vi "Periodic Tasks.vi"() -> ()   [LabVIEW 2011]
doc: "This VI runs in parallel to other tasks. It can contain as many user-defined periodic loops as you need. These can carry out PID or other sorts of timed response."
uses:
  <vilib>/Rock Robotics/WPI/Relay/WPI_RelayValue.ctl
  <vilib>/Rock Robotics/SystemInterfaces/Utilities/FPGA_UtilitiesLED State.ctl
  <vilib>/Rock Robotics/SystemInterfaces/Utilities/FPGA_UtilitiesLED Source.ctl
  Robot Global Data.vi
panel:
  out "Distance 2":dbl
  out "Direction 2":bool
  out "error out 3":errorcluster
  out "Rate 2":dbl
  out "Rate":dbl
  out "error out 2":errorcluster
  out "error out":errorcluster
  out "I2C":bool
  out "Heading 2":u16
  out "loop time":u32
  out "Angular Rate":dbl
  out "Angle":dbl
  out "Direction":bool
  out "Distance":dbl
  in  "Home Speed":dbl=1.0
  in  "Home Position":dbl=2.85
  out "Current Voltage":dbl
  in  "upper limit":dbl=4.5
  in  "lower limit":dbl=0.85
  # "Speed to move to home"
  # "Target Tracking"
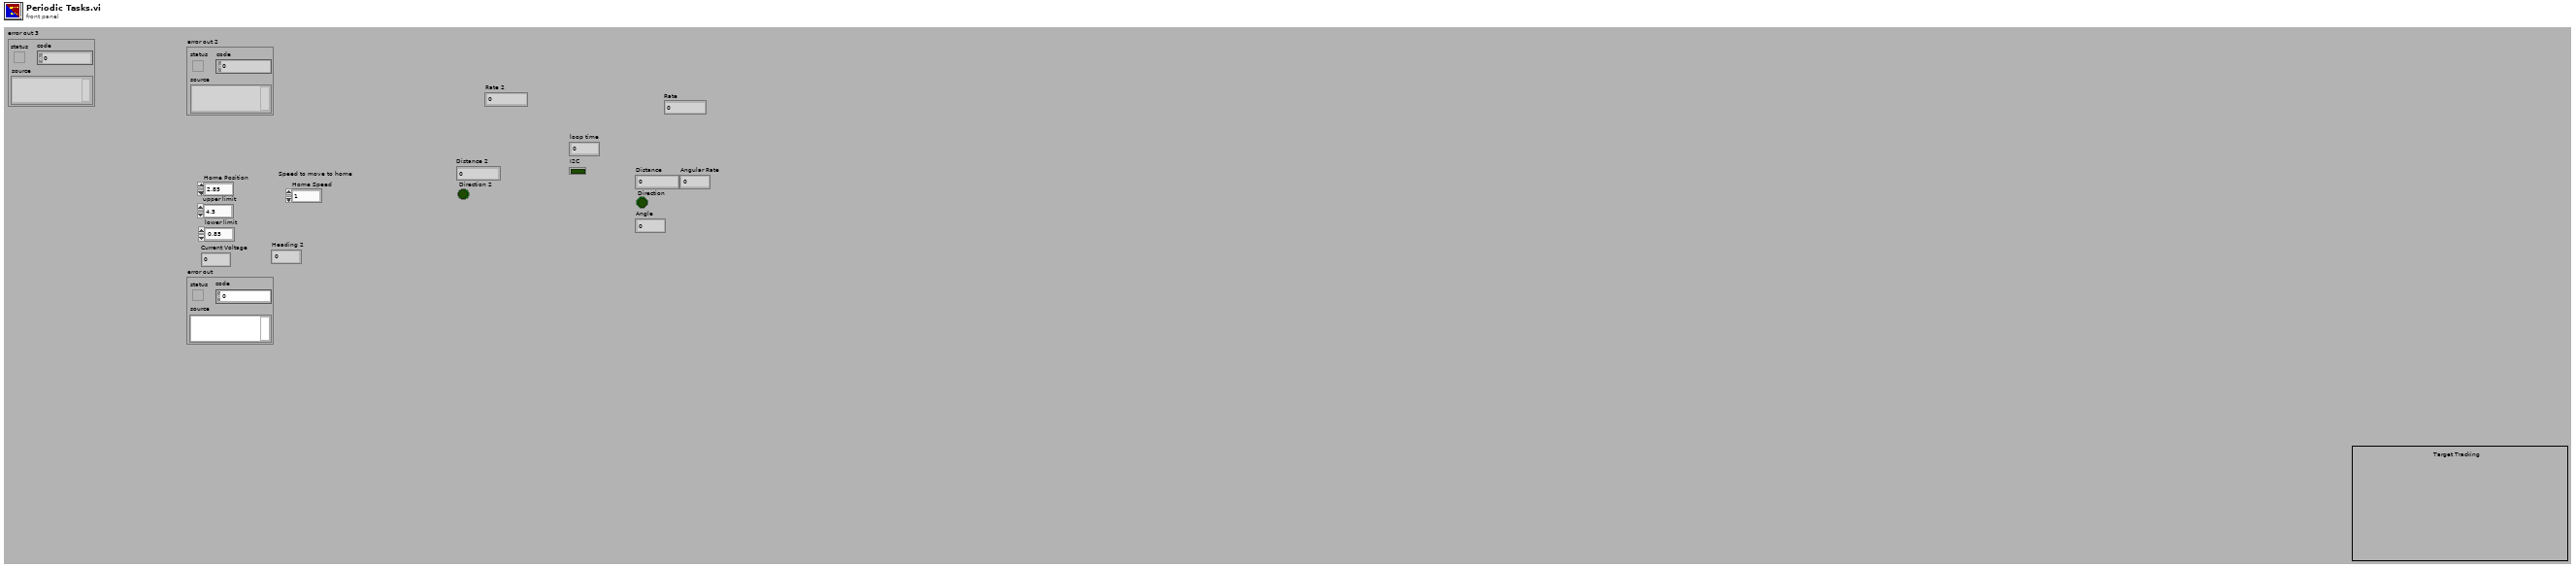
[diagram p1: front panel]
types:
  T1 = typedef "WPI_EncoderDevRef.ctl" = cluster{"DevStatus":errorcluster, "EncoderIndex":T2, "CounterIndex":T3, "DistancePerCount":dbl, "Decoding Type":T4}
  T2 = typedef "FPGA_EncoderIdx.ctl" = enum8{"Enc 0", "Enc 1", "Enc 2", "Enc 3", "Invalid"}
  T3 = typedef "FPGA_CounterCtrSystemIndex.ctl" = enum8{"Ctr 0", "Ctr 1", "Ctr 2", "Ctr 3", "Ctr 4", "Ctr 5", "Ctr 6", "Ctr 7", "Invalid"}
  T4 = typedef "WPI_EncoderType.ctl" = enum16{"1x", "2x", "4x"}
  T5 = typedef "WPI_RelayValue.ctl" = enum16{"Off", "On", "Forward", "Reverse"}
  T6 = typedef "WPI_GyroDevRef.ctl" = cluster{"DevStatus":errorcluster, "Analog Module":T7, "Analog Channel":T8, "Offset":dbl, "Gain (VoltsPerDegree/Second)":dbl}
  T7 = typedef "FPGA_TypedefAnalogModule.ctl" = enum16{"Analog Module 1", "Analog Module 2"}
  T8 = typedef "FPGA_AIChannel.ctl" = enum8{"AI 1", "AI 2", "AI 3", "AI 4", "AI 5", "AI 6", "AI 7", "AI 8", "Invalid"}
  T9 = typedef "WPI_I2CDevRef.ctl" = cluster{"DevStatus":errorcluster, "Digital Module":T10, "Device Address":u8}
  T10 = typedef "FPGA_TypedefDigitalModule.ctl" = enum16{"Digital Module 1", "Digital Module 2"}
  T11 = typedef "WPI_AnalogChannelDevRef.ctl" = cluster{"DevStatus":errorcluster, "Analog Module":T7, "Analog Channel":T8}
  T12 = typedef "WPI_RelayDevRef.ctl" = cluster{"DevStatus":errorcluster, "Relay Channel":T13, "Digital Module":T10, "Relay Direction":T14}
  T13 = typedef "FPGA_DIORelayChannel.ctl" = enum8{"Relay 1", "Relay 2", "Relay 3", "Relay 4", "Relay 5", "Relay 6", "Relay 7", "Relay 8", "Invalid"}
  T14 = typedef "WPI_RelayDirection.ctl" = enum16{"Both directions", "Forward only", "Reverse only"}
  T15 = cluster{"Driver Station Digital Output (1-8)[0]":bool, "Driver Station Digital Output (1-8)[1]":bool, "Driver Station Digital Output (1-8)[2]":bool, "Driver Station Digital Output (1-8)[3]":bool, "Driver Station Digital Output (1-8)[4]":bool, "Driver Station Digital Output (1-8)[5]":bool, "Driver Station Digital Output (1-8)[6]":bool, "Driver Station Digital Output (1-8)[7]":bool, "Driver Station Digital Output (1-8)[8]":bool}
  T16 = typedef "FPGA_UtilitiesLED State.ctl" = enum16{"Off", "On", "Toggle"}
  T17 = typedef "FPGA_UtilitiesLED Source.ctl" = enum16{"User LED", "FPGA LED"}
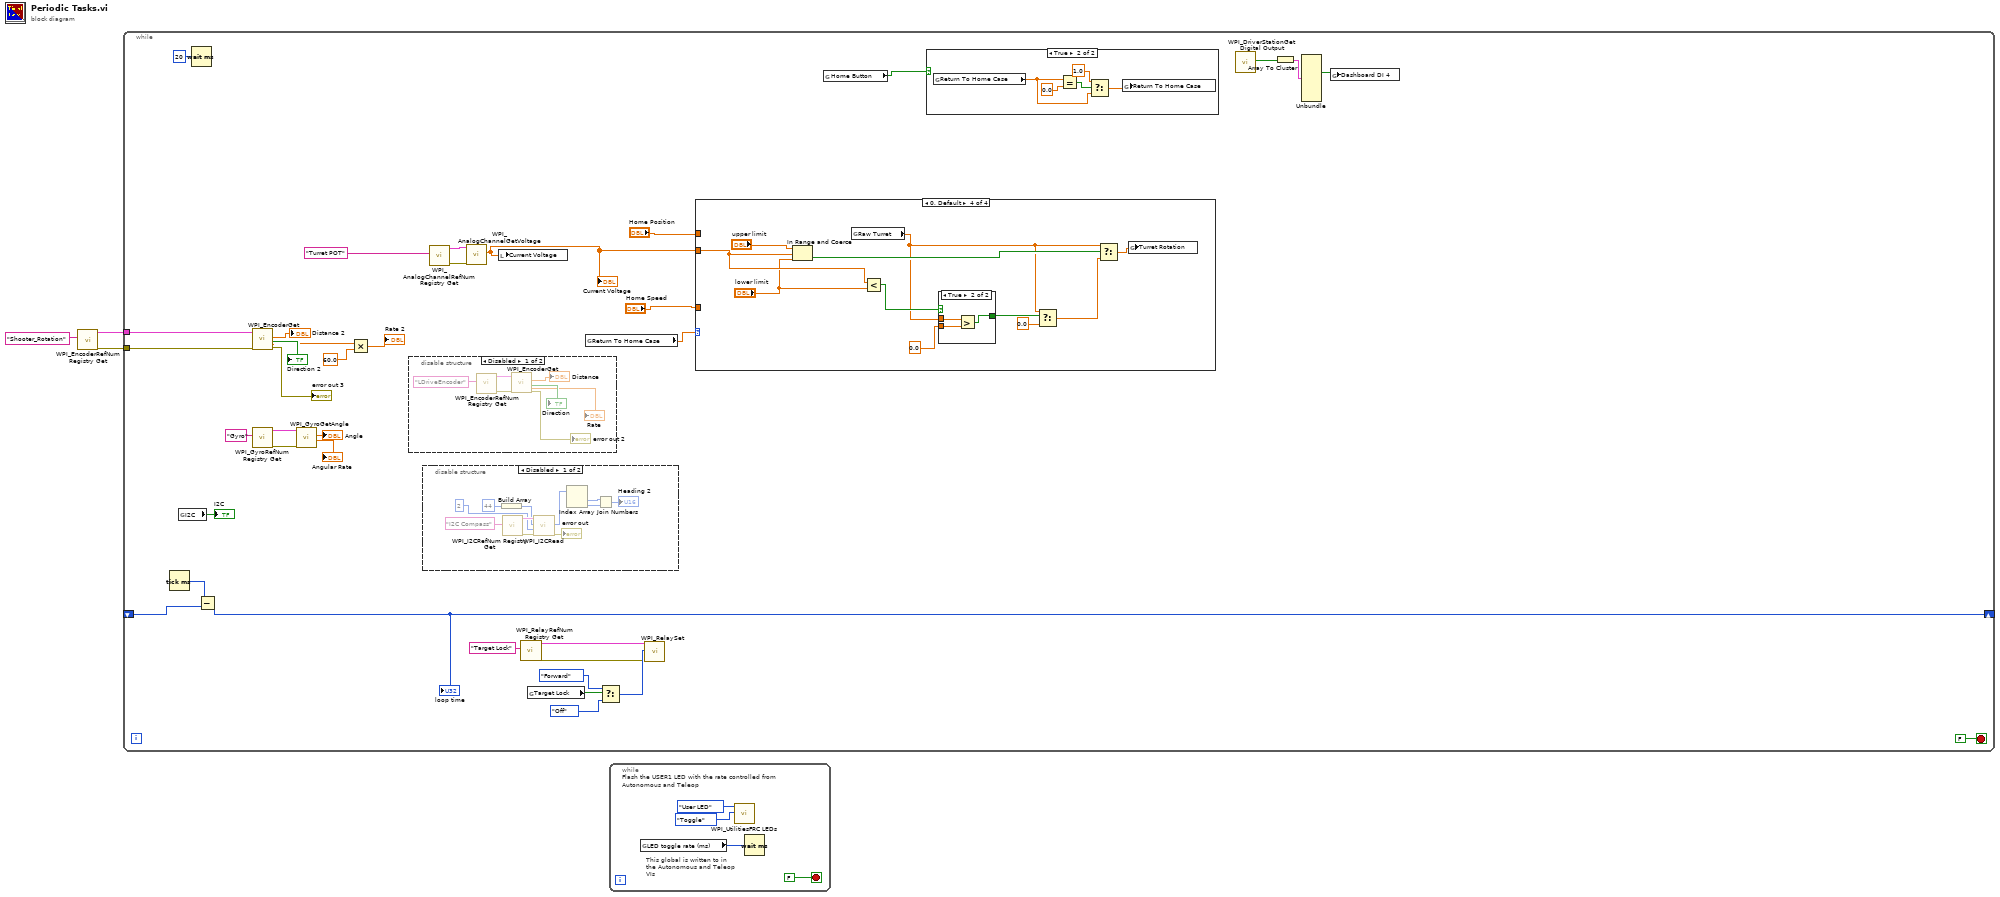
[diagram p0: block diagram]
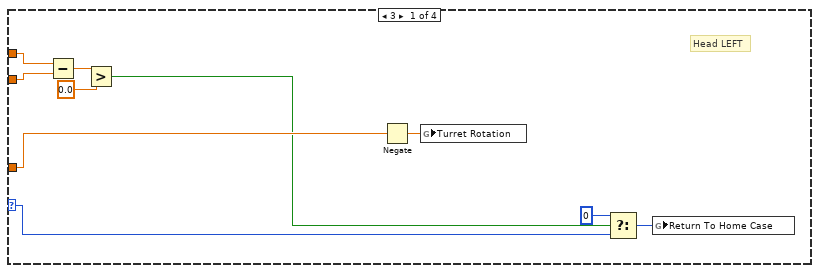
[diagram p4: hidden frame]
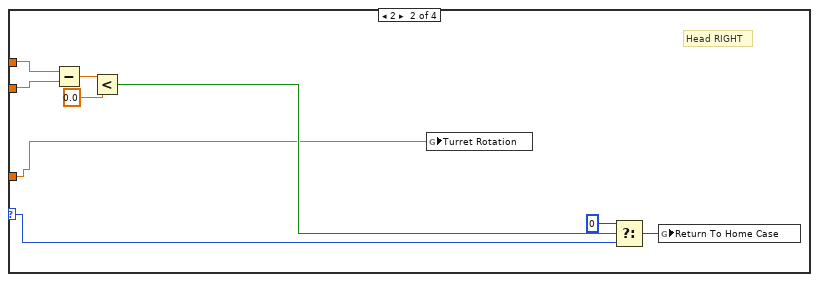
[diagram p5: hidden frame]
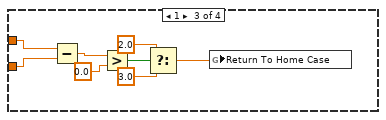
[diagram p6: hidden frame]
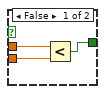
[diagram p7: hidden frame]
diagram:
  n1 = call <vilib>:"WPI_EncoderRefNum Registry Get.vi"("refnum name"="Shooter_Rotation") -> ("error out"=w2:errorcluster, "EncoderDevRef"=w1:T1)  [unwired: 9 in]
  n2 = while {
    shift-right: [w14] -> _
    shift-left: _ -> [w13]
    tunnel: w2 -> [w8]
    tunnel: w1 -> [w7]
    stop <- FALSE stop-if-true
    n3 = Tick Count (ms)() -> (millisecond timer value=w15:u32)
    n4 = global read "Robot Global Data.vi" "I2C"() -> (→"I2C":bool)
    n5 = Wait (ms)(milliseconds to wait=u32 20) -> ()  [unwired: 1 out]
    n6 = Subtract(x=w15, y=w13) -> (x-y=w14:u32)
    "loop time" <- w14
    n7 = call <vilib>:"WPI_EncoderGet.vi"("error in (no error)"=w8, "EncoderDevRef"=w7) -> ("error out"=→"error out 3":errorcluster, "Direction"=→"Direction 2":bool, "Distance"=→"Distance 2":dbl, "Rate"=w5:dbl)  [unwired: 4 in, 2 out]
    n8 = call <vilib>:"WPI_GyroRefNum Registry Get.vi"("refnum name"="Gyro") -> ("error out"=w19:errorcluster, "GyroDevRef"=w20:T6)  [unwired: 9 in]
    n9 = call <vilib>:"WPI_GyroGetAngle.vi"("error in (no error)"=w19, "GyroDevRef"=w20) -> ("Angular Rate"=→"Angular Rate":dbl, "Angle"=→"Angle":dbl)  [unwired: 6 in, 2 out]
    n10 = Multiply(x=w5, y=60.0) -> (x*y=→"Rate 2":dbl)
    n11 = disable-structure shown="Disabled" {
      frame Disabled {
        n12 = call <vilib>:"WPI_EncoderRefNum Registry Get.vi"("refnum name"="LDriveEncoder") -> ("error out"=w55:errorcluster, "EncoderDevRef"=w56:T1)  [unwired: 9 in]
        n13 = call <vilib>:"WPI_EncoderGet.vi"("error in (no error)"=w55, "EncoderDevRef"=w56) -> ("error out"=→"error out 2":errorcluster, "Direction"=→"Direction":bool, "Distance"=→"Distance":dbl, "Rate"=→"Rate":dbl)  [unwired: 4 in, 2 out]
      }
      frame Enabled {
      }
    }
    n14 = disable-structure shown="Disabled" {
      frame Disabled {
        n15 = Build Array(u8 44 ("element")) -> (w45:u8[])
        n16 = call <vilib>:"WPI_I2CRefNum Registry Get.vi"("refnum name"="I2C Compass") -> ("error out"=w51:errorcluster, "I2CDevRef"=w50:T9)  [unwired: 9 in]
        n17 = call <vilib>:"WPI_I2CRead.vi"("error in (no error)"=w51, "I2CBytesToRead"=u8 2, "I2CRegister"=w45, "I2CDevRef"=w50) -> ("error out"=→"error out":errorcluster, "Data Out"=w49:u8[])  [unwired: 5 in, 1 out]
        n18 = Index Array(array=w49) -> (element #1=w47:u8, element #2=w48:u8)  [unwired: 2 in]
        n19 = Join Numbers(hi=w47, lo=w48) -> ((hi.lo)=→"Heading 2":u16)
      }
      frame Enabled {
      }
    }
    n20 = call <vilib>:"WPI_AnalogChannelRefNum Registry Get.vi"("refnum name"="Turret POT") -> ("error out"=w21:errorcluster, "AIDeviceRef"=w22:T11)  [unwired: 9 in]
    n21 = call <vilib>:"WPI_AnalogChannelGetVoltage.vi"("error in (no error)"=w21, "AIDeviceRef"=w22) -> ("Voltage"=w29:dbl)  [unwired: 7 in, 2 out]
    "Current Voltage" <- w29
    n22 = local write "Current Voltage"(w29) -> ()
    n23 = call <vilib>:"WPI_RelayRefNum Registry Get.vi"("refnum name"="Target Lock") -> ("error out"=w31:errorcluster, "RelayDevRef"=w32:T12)  [unwired: 9 in]
    n24 = global read "Robot Global Data.vi" "Target Lock"() -> (w37:bool)
    n25 = global read "Robot Global Data.vi" "Return To Home Case"() -> (w28:dbl)
    n26 = Select(t=WPI_RelayValue."Forward" ("RelayValue"), s=w37, f=WPI_RelayValue."Off" ("RelayValue")) -> (s? t:f=w34:T5)
    n27 = call <vilib>:"WPI_RelaySet.vi"("error in (no error)"=w31, "RelayValue"=w34, "RelayDevRef"=w32) -> ()  [unwired: 7 in, 2 out]
    n28 = case shown="0, Default" w28 {
      selector: w28 -> [w66 w70 _ _]
      tunnel: w29 -> [w62 w71 w84 w96]
      tunnel: "Home Position" -> [w63 w72 w85 _]
      tunnel: "Home Speed" -> [w64 w69 _ _]
      frame 3 {
        # "Head LEFT"
        n29 = Subtract(x=w63, y=w62) -> (x-y=w61:dbl)
        n30 = Greater?(x=w61, y=0.0) -> (0:w59:bool)
        n31 = Negate(x=w64) -> (-x=w65:dbl)
        n32 = global write "Robot Global Data.vi" "Turret Rotation"(w65) -> ()
        n33 = Select(t=0, s=w59, f=w66) -> (s? t:f=w67:i32)
        n34 = global write "Robot Global Data.vi" "Return To Home Case"(w67) -> ()
      }
      frame 2 {
        # "Head RIGHT"
        n35 = Subtract(x=w72, y=w71) -> (x-y=w75:dbl)
        n36 = Less?(x=w75, y=0.0) -> (x < y?=w73:bool)
        n37 = global write "Robot Global Data.vi" "Turret Rotation"(w69) -> ()
        n38 = Select(t=0, s=w73, f=w70) -> (s? t:f=w76:i32)
        n39 = global write "Robot Global Data.vi" "Return To Home Case"(w76) -> ()
      }
      frame 1 {
        n40 = Subtract(x=w85, y=w84) -> (x-y=w83:dbl)
        n41 = Greater?(x=w83, y=0.0) -> (0:w81:bool)
        n42 = Select(t=2.0, s=w81, f=3.0) -> (s? t:f=w78:dbl)
        n43 = global write "Robot Global Data.vi" "Return To Home Case"(w78) -> ()
      }
      frame 0, Default {
        n44 = In Range and Coerce(upper limit="upper limit", x=w96, lower limit="lower limit") -> (In Range?=w93:bool)  [unwired: 1 out]
        n45 = global read "Robot Global Data.vi" "Raw Turret"() -> (w86:dbl)
        n46 = Less?(x=w96, y="lower limit") -> (x < y?=w88:bool)
        n47 = case shown="True" w88 {
          tunnel: 0.0 -> [w98 w102]
          tunnel: [w97 w101] -> w89
          tunnel: w86 -> [w99 w100]
          frame False {
            n48 = Less?(x=w99, y=w98) -> (x < y?=w97:bool)
          }
          frame True {
            n49 = Greater?(x=w100, y=w102) -> (0:w101:bool)
          }
        }
        n50 = Select(t=w86, s=w89, f=0.0) -> (s? t:f=w87:dbl)
        n51 = Select(t=w86, s=w93, f=w87) -> (s? t:f=w95:dbl)
        n52 = global write "Robot Global Data.vi" "Turret Rotation"(w95) -> ()
      }
    }
    n53 = global read "Robot Global Data.vi" "Home Button"() -> (w25:bool)
    n54 = case shown="True" w25 {
      frame False {
      }
      frame True {
        n55 = global read "Robot Global Data.vi" "Return To Home Case"() -> (w104:dbl)
        n56 = Equal?(x=w104, y=0.0) -> (x = y?=w106:bool)
        n57 = Select(t=1.0, s=w106, f=w104) -> (s? t:f=w103:dbl)
        n58 = global write "Robot Global Data.vi" "Return To Home Case"(w103) -> ()
      }
    }
    n59 = call <vilib>:"WPI_DriverStationGet Digital Output.vi"() -> ("Driver Station Digital Output (1-8)"=w40:bool[])  [unwired: 10 in, 1 out]
    n60 = Array To Cluster(array=w40) -> (cluster=w39:T15)
    n61 = Unbundle(w39) -> ("Driver Station Digital Output (1-8)[3]"=w38:bool)  [unwired: 8 out]
    n62 = global write "Robot Global Data.vi" "Dashboard DI 4"(w38) -> ()
  }
  n63 = while {
    stop <- FALSE stop-if-true
    # "This global is written to in the Autonomous and Teleop VIs"
    # "Flash the USER1 LED with the rate controlled from Autonomous and Teleop"
    n64 = global read "Robot Global Data.vi" "LED toggle rate (ms)"() -> (w108:u32)
    n65 = call <vilib>:"WPI_UtilitiesFRC LEDs.vi"("State"=FPGA_UtilitiesLED_State."Toggle", "LED Type"=FPGA_UtilitiesLED_Source."User LED") -> ()  [unwired: 1 in, 9 out]
    n66 = Wait (ms)(milliseconds to wait=w108) -> ()  [unwired: 1 out]
  }
